vi "Write generate report.vi"(0 "report in":refnum<class "NI_report.lvclass">, 7 "generate report":T1={"font"={"font name"="", "font size"=0.0, "bold"=0, "italic"=0, "underline"=0, "strike through"=0, "font color"=16777216}, "from template?"=FALSE} {"font"."font size" format="%0.2f"; "font"."strike through" items=["Unchanged", "Yes", "No"]; "font"."underline" items=["Unchanged", "Yes", "No"]; "font"."italic" items=["Unchanged", "Yes", "No"]; "font"."bold" items=["Unchanged", "Yes", "No"]}, 11 "error in (no error)":errorcluster) -> (4 "report out":refnum<class "NI_report.lvclass">, 15 "error out":errorcluster)   [LabVIEW 2020, in "NI_report.lvclass"]
uses:
  NI_report.lvclass
  Report Data Members.ctl
  font.ctl
  NI_report.lvclass/NI_report.ctl
  NI_ReportGenerationCore.lvlib
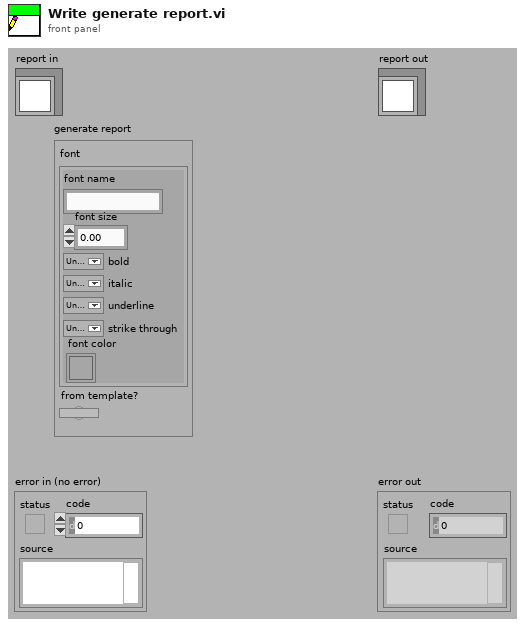
[diagram p1: front panel]
types:
  T1 = typedef "NI_ReportGenerationCore.lvlib/Report Data Members.ctl" = cluster{"font":T2, "from template?":bool}
  T2 = typedef "NI_ReportGenerationCore.lvlib/font.ctl" = cluster{"font name":string, "font size":dbl, "bold":u16, "italic":u16, "underline":u16, "strike through":u16, "font color":u32}
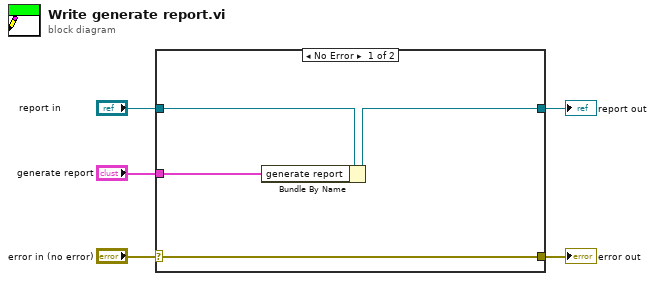
[diagram p0: block diagram]
diagram:
  n1 = case shown="No Error" "error in (no error)" {
    selector: "error in (no error)" -> [w9 w10]
    tunnel: [w9 w10] -> w4
    tunnel: [w7 w11] -> w2
    tunnel: "report in" -> [w8 w11]
    tunnel: "generate report" -> [w6 _]
    frame No Error {
      n2 = Bundle By Name(cluster=w8, "generate report"=w6) -> (w7:refnum<class "NI_report.lvclass">)
    }
    frame Error {
    }
  }
  "error out" <- w4
  "report out" <- w2
